vi "Simple Add.vi"(10 "y":dbl format="%#_13g", 11 "x":dbl format="%#_13g") -> (3 "sum":dbl)   [LabVIEW 2018]
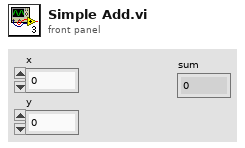
[diagram p1: front panel]
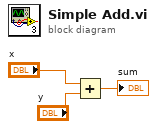
[diagram p0: block diagram]
diagram:
  n1 = Add(x="x", y="y") -> (x+y=→"sum":dbl)
